vi "V Function.vi"(1 "H input":dbl, 2 "Z input":dbl, 3 "Y input":dbl, 4 "Max Velocity":dbl) -> (0 "V":dbl)   [LabVIEW 2012]
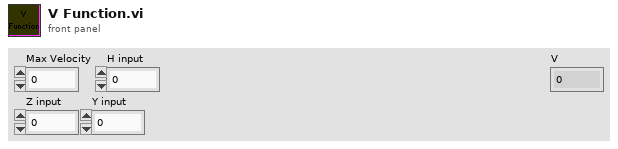
[diagram p1: front panel]
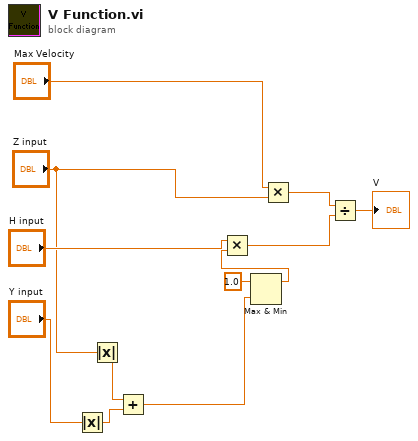
[diagram p0: block diagram]
diagram:
  n1 = Absolute Value(x="Y input") -> (abs(x)=w7:dbl)
  n2 = Absolute Value(x="Z input") -> (abs(x)=w6:dbl)
  n3 = Add(x=w6, y=w7) -> (x+y=w3:dbl)
  n4 = Max & Min(x=1.0, y=w3) -> (max(x,y)=w9:dbl)  [unwired: 1 out]
  n5 = Multiply(x="H input", y=w9) -> (x*y=w2:dbl)
  n6 = Multiply(x="Max Velocity", y="Z input") -> (x*y=w11:dbl)
  n7 = Divide(x=w11, y=w2) -> (x/y=→"V":dbl)
